vi "Create IO Channels Parallel.vi"(6 "AI Buffer Size (s)":i32=10, 8 "AI Block Size":i32=5000, 9 "Cluster":T1={"amplitude (V)"=[0.001, 2e-08, 0.001, 0.001, 0.001, 2e-08, 0.0, 0.0], "DC (V)"=[0.0, 0.0, 0.0, 0.0, 0.0, 0.0, 0.0, 0.0], "f (Hz)"=[13.0, 13.0, 13.0, 13.0, 13.0, 13.0, 13.0, 13.0], "phase (deg)"=[0.0, 0.0, 0.0, 0.0, 0.0, 0.0, 0.0, 0.0], "demod f (Hz)"=[13.0, 13.0, 13.0, 13.0, 13.0, 13.0, 13.0, 13.0], "function"=[enum."Sine Wave", enum."Sine Wave", enum."Sine Wave", enum."Sine Wave", enum."Sine Wave", enum."Sine Wave", enum."Sine Wave", enum."Sine Wave"]} {"DC (V)" format="%#_6p"; "amplitude (V)" format="%#_6p"}, 10 "AO Configuration":T2(array[cluster])=[{"Output physical channels"="PXI1Slot2/ao0", "AO. Max"=0.1, "AO.Min"=-0.1}, {"Output physical channels"="", "AO. Max"=0.1, "AO.Min"=-0.1}], 11 "AI Configuration":T3(array[cluster])=[{"AI.Coupling"=10050, "AI.Max"=10.0, "AI.Min"=-10.0, "Input physical channels"="PXI1Slot2/ai0:1"}, {"AI.Coupling"=10050, "AI.Max"=10.0, "AI.Min"=-10.0, "Input physical channels"="PXI1Slot3/ai0:3"}, {"AI.Coupling"=10050, "AI.Max"=10.0, "AI.Min"=-10.0, "Input physical channels"=""}] {"AI.Coupling" items=["AC"=10045, "DC"=10050, "GND"=10066]}) -> (0 "sampling info":cluster{"Fs":dbl, "#s":dbl}, 1 "AI Rate":dbl=10000.0 format="%.2f", 2 "AO Task":refnum<k21>[](array[refnum]), 3 "AI task":refnum<k21>[](array[refnum]), 4 "phase log":dbl[](array[numeric])=[0.99999999999938, 0.99999999999938], 5 "appended array":errorcluster[][](array[cluster]))   [LabVIEW 2013]
uses:
  <vilib>/DAQmx/write.llb/DAQmx Write (Analog 1D Wfm NChan NSamp).vi
  <vilib>/DAQmx/create/channels.llb/DAQmx Create Channel (AI-Voltage-Basic).vi
  <vilib>/DAQmx/create/channels.llb/DAQmx Create Channel (AO-Voltage-Basic).vi
  <vilib>/DAQmx/configure/timing.llb/DAQmx Timing (Sample Clock).vi
  <vilib>/DAQmx/configure/trigger.llb/DAQmx Start Trigger (Digital Edge).vi
  <vilib>/DAQmx/miscellaneous.llb/DAQmx Fill In Error Info.vi
  <resource>/objmgr/daqmx.rc
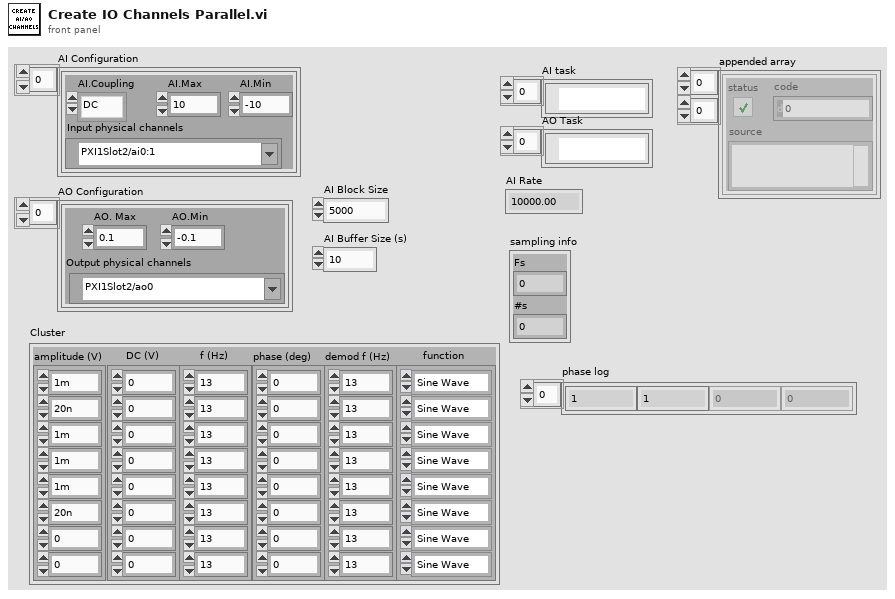
[diagram p1: front panel]
types:
  T1 = cluster{"amplitude (V)":dbl[], "DC (V)":dbl[], "f (Hz)":dbl[], "phase (deg)":dbl[], "demod f (Hz)":dbl[], "function":enum16{"Sine Wave", "Triangle Wave", "Square Wave", "Sawtooth Wave"}[]}
  T2 = cluster{"Output physical channels":tag, "AO. Max":dbl, "AO.Min":dbl}[]
  T3 = cluster{"AI.Coupling":i32, "AI.Max":dbl, "AI.Min":dbl, "Input physical channels":tag}[]
  T4 = cluster{"AI.Coupling":i32, "AI.Max":dbl, "AI.Min":dbl, "Input physical channels":tag}
  T5 = cluster{"Output physical channels":tag, "AO. Max":dbl, "AO.Min":dbl}
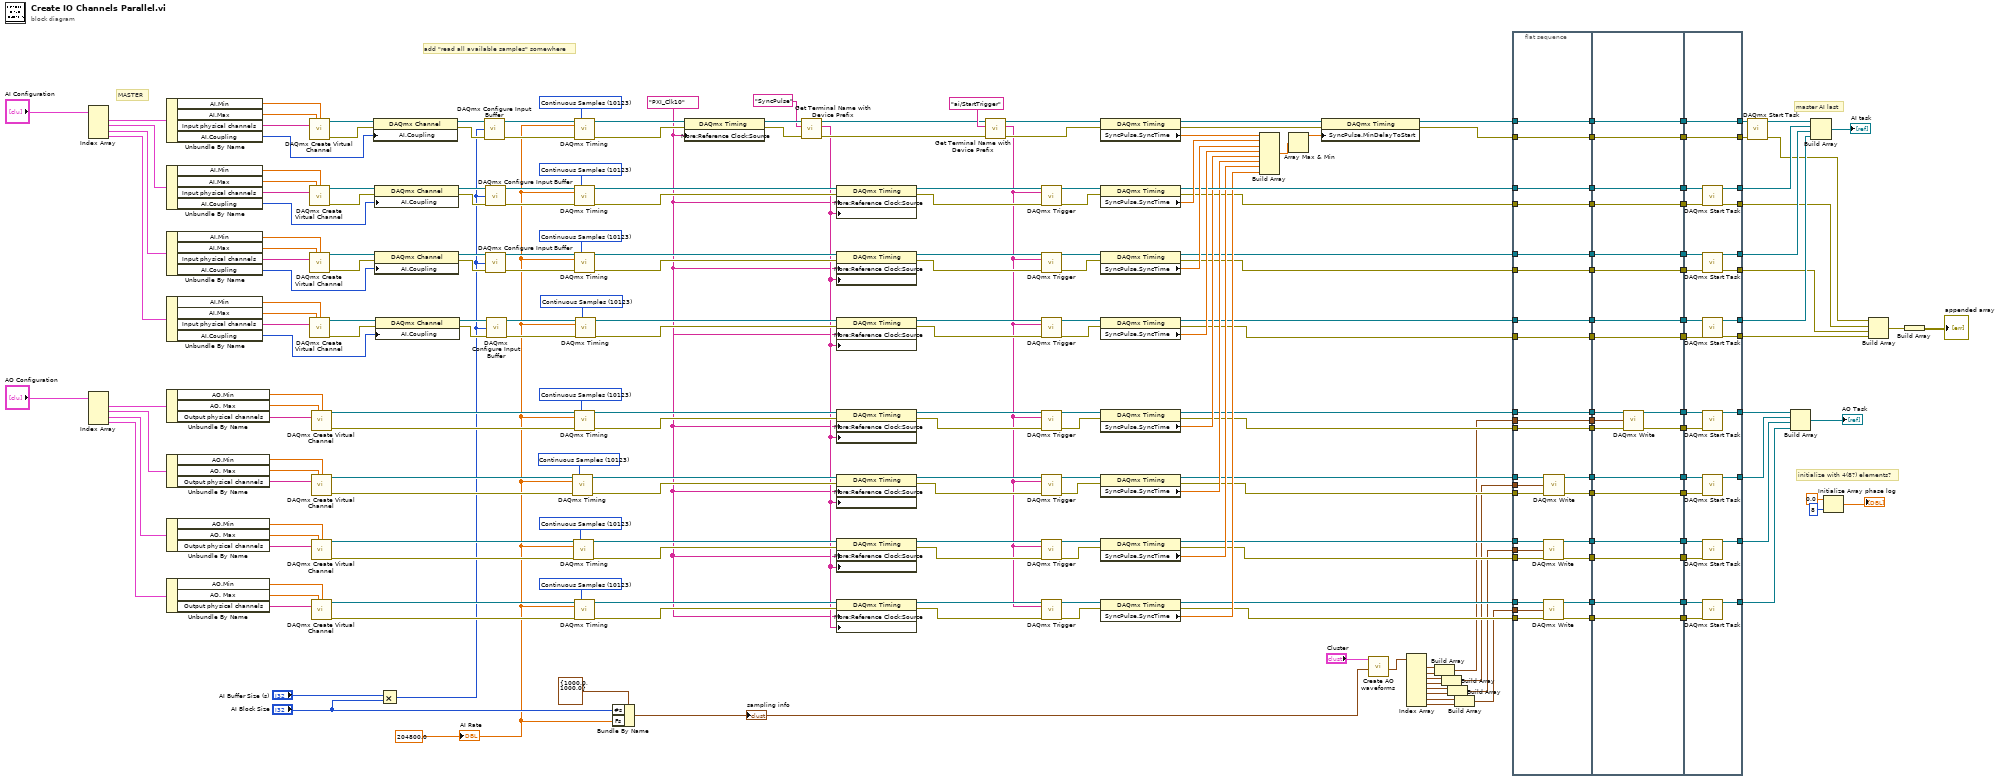
[diagram p0: block diagram]
diagram:
  w7 = 204800.0
  w23 = tag "PXI_Clk10" ("RefClk.Src")
  w96 = 10123 items=["Finite Samples"=10178, "Continuous Samples"=10123] ("sample mode")
  w111 = 10123 items=["Finite Samples"=10178, "Continuous Samples"=10123] ("sample mode")
  w120 = 10123 items=["Finite Samples"=10178, "Continuous Samples"=10123] ("sample mode")
  w134 = 10123 items=["Finite Samples"=10178, "Continuous Samples"=10123] ("sample mode")
  w161 = 10123 items=["Finite Samples"=10178, "Continuous Samples"=10123] ("sample mode")
  w177 = 10123 items=["Finite Samples"=10178, "Continuous Samples"=10123] ("sample mode")
  w190 = 10123 items=["Finite Samples"=10178, "Continuous Samples"=10123] ("sample mode")
  w230 = 10123 items=["Finite Samples"=10178, "Continuous Samples"=10123] ("sample mode")
  # "master AI last"
  # "initialize with 4(8?) elements?"
  # "add \"read all available samples\" somewhere"
  # "MASTER"
  n1 = Index Array(array="AI Configuration") -> (element #1=w231:T4, element #2=w191:T4, element #3=w154:T4, element #4=w153:T4)  [unwired: 4 in]
  n2 = Index Array(array="AO Configuration") -> (element #1=w138:T5, element #2=w89:T5, element #3=w90:T5, element #4=w91:T5)  [unwired: 4 in]
  n3 = Unbundle By Name(w231) -> ("AI.Min"=w202:dbl, "AI.Max"=w203:dbl, "Input physical channels"=w215:tag, "AI.Coupling"=w201:i32)
  n4 = Unbundle By Name(w191) -> ("AI.Min"=w198:dbl, "AI.Max"=w197:dbl, "Input physical channels"=w192:tag, "AI.Coupling"=w199:i32)
  n5 = Unbundle By Name(w154) -> ("AI.Min"=w170:dbl, "AI.Max"=w171:dbl, "Input physical channels"=w176:tag, "AI.Coupling"=w169:i32)
  n6 = Unbundle By Name(w153) -> ("AI.Min"=w167:dbl, "AI.Max"=w166:dbl, "Input physical channels"=w162:tag, "AI.Coupling"=w168:i32)
  n7 = Unbundle By Name(w138) -> ("AO.Min"=w135:dbl, "AO. Max"=w136:dbl, "Output physical channels"=w137:tag)
  n8 = Unbundle By Name(w89) -> ("AO.Min"=w118:dbl, "AO. Max"=w117:dbl, "Output physical channels"=w116:tag)
  n9 = Unbundle By Name(w90) -> ("AO.Min"=w113:dbl, "AO. Max"=w114:dbl, "Output physical channels"=w115:tag)
  n10 = Unbundle By Name(w91) -> ("AO.Min"=w94:dbl, "AO. Max"=w93:dbl, "Output physical channels"=w92:tag)
  n11 = call-poly <vilib>:"DAQmx Create Virtual Channel.vi"("maximum value"=w203, "minimum value"=w202, "physical channels"=w215) -> ("task out"=w214:refnum<k21>, "error out"=w213:errorcluster)  [unwired: 11 in]
  n12 = call-poly <vilib>:"DAQmx Create Virtual Channel.vi"("maximum value"=w197, "minimum value"=w198, "physical channels"=w192) -> ("task out"=w193:refnum<k21>, "error out"=w194:errorcluster)  [unwired: 11 in]
  n13 = call-poly <vilib>:"DAQmx Create Virtual Channel.vi"("maximum value"=w171, "minimum value"=w170, "physical channels"=w176) -> ("task out"=w175:refnum<k21>, "error out"=w174:errorcluster)  [unwired: 11 in]
  n14 = call-poly <vilib>:"DAQmx Create Virtual Channel.vi"("maximum value"=w166, "minimum value"=w167, "physical channels"=w162) -> ("task out"=w163:refnum<k21>, "error out"=w164:errorcluster)  [unwired: 11 in]
  n15 = call-poly <vilib>:"DAQmx Create Virtual Channel.vi"("maximum value"=w136, "minimum value"=w135, "physical channels"=w137) -> ("task out"=w21:refnum<k21>, "error out"=w20:errorcluster)  [unwired: 11 in]
  n16 = call-poly <vilib>:"DAQmx Create Virtual Channel.vi"("maximum value"=w117, "minimum value"=w118, "physical channels"=w116) -> ("task out"=w119:refnum<k21>, "error out"=w121:errorcluster)  [unwired: 11 in]
  n17 = call-poly <vilib>:"DAQmx Create Virtual Channel.vi"("maximum value"=w114, "minimum value"=w113, "physical channels"=w115) -> ("task out"=w112:refnum<k21>, "error out"=w110:errorcluster)  [unwired: 11 in]
  n18 = call-poly <vilib>:"DAQmx Create Virtual Channel.vi"("maximum value"=w93, "minimum value"=w94, "physical channels"=w92) -> ("task out"=w95:refnum<k21>, "error out"=w97:errorcluster)  [unwired: 11 in]
  n19 = property class="DAQmx Channel"(reference=w214, error in=w213, "AI.Coupling"=w201) -> (reference out=w212:refnum<k21>, error out=w211:errorcluster)
  n20 = property class="DAQmx Channel"(reference=w193, error in=w194, "AI.Coupling"=w199) -> (reference out=w195:refnum<k21>, error out=w196:errorcluster)
  n21 = property class="DAQmx Channel"(reference=w175, error in=w174, "AI.Coupling"=w169) -> (reference out=w173:refnum<k21>, error out=w172:errorcluster)
  n22 = property class="DAQmx Channel"(reference=w163, error in=w164, "AI.Coupling"=w168) -> (reference out=w165:refnum<k21>, error out=w28:errorcluster)
  n23 = Multiply(x="AI Buffer Size (s)", y="AI Block Size") -> (x*y=w4:i32)
  n24 = call <vilib>:"DAQmx Configure Input Buffer.vi"("task/channels in"=w212, "buffer size (in samples per channel)"=w4, "error in"=w211) -> ("task out"=w210:refnum<k21>, "error out"=w209:errorcluster)  [unwired: 11 in]
  n25 = call <vilib>:"DAQmx Configure Input Buffer.vi"("task/channels in"=w195, "buffer size (in samples per channel)"=w4, "error in"=w196) -> ("task out"=w189:refnum<k21>, "error out"=w188:errorcluster)  [unwired: 11 in]
  n26 = call <vilib>:"DAQmx Configure Input Buffer.vi"("task/channels in"=w173, "buffer size (in samples per channel)"=w4, "error in"=w172) -> ("task out"=w178:refnum<k21>, "error out"=w179:errorcluster)  [unwired: 11 in]
  n27 = call <vilib>:"DAQmx Configure Input Buffer.vi"("task/channels in"=w165, "buffer size (in samples per channel)"=w4, "error in"=w28) -> ("task out"=w160:refnum<k21>, "error out"=w159:errorcluster)  [unwired: 11 in]
  n28 = call-poly <vilib>:"DAQmx Timing.vi"("task/channels in"=w119, "sample mode"=w120, "rate"=w7, "error in"=w121) -> ("task out"=w123:refnum<k21>, "error out"=w124:errorcluster)  [unwired: 10 in]
  n29 = call-poly <vilib>:"DAQmx Timing.vi"("task/channels in"=w112, "sample mode"=w111, "rate"=w7, "error in"=w110) -> ("task out"=w108:refnum<k21>, "error out"=w107:errorcluster)  [unwired: 10 in]
  n30 = call-poly <vilib>:"DAQmx Timing.vi"("task/channels in"=w210, "sample mode"=w230, "rate"=w7, "error in"=w209) -> ("task out"=w229:refnum<k21>, "error out"=w200:errorcluster)  [unwired: 10 in]
  n31 = call-poly <vilib>:"DAQmx Timing.vi"("task/channels in"=w189, "sample mode"=w190, "rate"=w7, "error in"=w188) -> ("task out"=w187:refnum<k21>, "error out"=w186:errorcluster)  [unwired: 10 in]
  n32 = call-poly <vilib>:"DAQmx Timing.vi"("task/channels in"=w178, "sample mode"=w177, "rate"=w7, "error in"=w179) -> ("task out"=w180:refnum<k21>, "error out"=w181:errorcluster)  [unwired: 10 in]
  n33 = call-poly <vilib>:"DAQmx Timing.vi"("task/channels in"=w21, "sample mode"=w134, "rate"=w7, "error in"=w20) -> ("task out"=w132:refnum<k21>, "error out"=w131:errorcluster)  [unwired: 10 in]
  n34 = call-poly <vilib>:"DAQmx Timing.vi"("task/channels in"=w95, "sample mode"=w96, "rate"=w7, "error in"=w97) -> ("task out"=w99:refnum<k21>, "error out"=w100:errorcluster)  [unwired: 10 in]
  n35 = call-poly <vilib>:"DAQmx Timing.vi"("task/channels in"=w160, "sample mode"=w161, "rate"=w7, "error in"=w159) -> ("task out"=w158:refnum<k21>, "error out"=w157:errorcluster)  [unwired: 10 in]
  n36 = Bundle By Name(cluster=cluster{"Fs":dbl, "#s":dbl} {"Fs"=1000.0, "#s"=1000.0} ("sampling info"), "#s"="AI Block Size", "Fs"=w7) -> (w6:cluster{"Fs":dbl, "#s":dbl})
  "sampling info" <- w6
  n37 = property class="DAQmx Timing"(reference=w229, error in=w200, "More:Reference Clock:Source"=w23) -> (reference out=w27:refnum<k21>, error out=w26:errorcluster)
  n38 = call "Get Terminal Name with Device Prefix.vi"("error in (no error)"=w26, "Local Terminal Name"="SyncPulse", "task/channels in"=w27) -> ("error out"=w224:errorcluster, "Terminal Name with Device Prefix"=w24:tag, "task out"=w225:refnum<k21>)  [unwired: 6 in]
  n39 = property class="DAQmx Timing"(reference=w187, error in=w186, "More:Reference Clock:Source"=w23, "More:Synchronization Pulse:Source"=w24) -> (reference out=w185:refnum<k21>, error out=w184:errorcluster)
  n40 = property class="DAQmx Timing"(reference=w180, error in=w181, "More:Reference Clock:Source"=w23, "More:Synchronization Pulse:Source"=w24) -> (reference out=w182:refnum<k21>, error out=w183:errorcluster)
  n41 = property class="DAQmx Timing"(reference=w158, error in=w157, "More:Reference Clock:Source"=w23, "More:Synchronization Pulse:Source"=w24) -> (reference out=w156:refnum<k21>, error out=w155:errorcluster)
  n42 = property class="DAQmx Timing"(reference=w132, error in=w131, "More:Reference Clock:Source"=w23, "More:Synchronization Pulse:Source"=w24) -> (reference out=w133:refnum<k21>, error out=w130:errorcluster)
  n43 = property class="DAQmx Timing"(reference=w123, error in=w124, "More:Reference Clock:Source"=w23, "More:Synchronization Pulse:Source"=w24) -> (reference out=w122:refnum<k21>, error out=w125:errorcluster)
  n44 = property class="DAQmx Timing"(reference=w108, error in=w107, "More:Reference Clock:Source"=w23, "More:Synchronization Pulse:Source"=w24) -> (reference out=w109:refnum<k21>, error out=w106:errorcluster)
  n45 = property class="DAQmx Timing"(reference=w99, error in=w100, "More:Reference Clock:Source"=w23, "More:Synchronization Pulse:Source"=w24) -> (reference out=w98:refnum<k21>, error out=w101:errorcluster)
  n46 = call "Get Terminal Name with Device Prefix.vi"("error in (no error)"=w224, "Local Terminal Name"="ai/StartTrigger", "task/channels in"=w225) -> ("error out"=w222:errorcluster, "Terminal Name with Device Prefix"=w84:tag, "task out"=w223:refnum<k21>)  [unwired: 6 in]
  n47 = call-poly <vilib>:"DAQmx Trigger.vi"("task/channels in"=w185, "source"=w84, "error in"=w184) -> ("task out"=w150:refnum<k21>, "error out"=w149:errorcluster)  [unwired: 11 in]
  n48 = call-poly <vilib>:"DAQmx Trigger.vi"("task/channels in"=w182, "source"=w84, "error in"=w183) -> ("task out"=w151:refnum<k21>, "error out"=w148:errorcluster)  [unwired: 11 in]
  n49 = call-poly <vilib>:"DAQmx Trigger.vi"("task/channels in"=w156, "source"=w84, "error in"=w155) -> ("task out"=w152:refnum<k21>, "error out"=w147:errorcluster)  [unwired: 11 in]
  n50 = call-poly <vilib>:"DAQmx Trigger.vi"("task/channels in"=w133, "source"=w84, "error in"=w130) -> ("task out"=w129:refnum<k21>, "error out"=w128:errorcluster)  [unwired: 11 in]
  n51 = call-poly <vilib>:"DAQmx Trigger.vi"("task/channels in"=w122, "source"=w84, "error in"=w125) -> ("task out"=w126:refnum<k21>, "error out"=w127:errorcluster)  [unwired: 11 in]
  n52 = call-poly <vilib>:"DAQmx Trigger.vi"("task/channels in"=w109, "source"=w84, "error in"=w106) -> ("task out"=w105:refnum<k21>, "error out"=w104:errorcluster)  [unwired: 11 in]
  n53 = call-poly <vilib>:"DAQmx Trigger.vi"("task/channels in"=w98, "source"=w84, "error in"=w101) -> ("task out"=w102:refnum<k21>, "error out"=w103:errorcluster)  [unwired: 11 in]
  n54 = property class="DAQmx Timing"(reference=w223, error in=w222) -> (reference out=w219:refnum<k21>, error out=w220:errorcluster, "SyncPulse.SyncTime"=w221:dbl)
  n55 = property class="DAQmx Timing"(reference=w150, error in=w149) -> (reference out=w140:refnum<k21>, error out=w75:errorcluster, "SyncPulse.SyncTime"=w145:dbl)
  n56 = property class="DAQmx Timing"(reference=w151, error in=w148) -> (reference out=w81:refnum<k21>, error out=w72:errorcluster, "SyncPulse.SyncTime"=w144:dbl)
  n57 = property class="DAQmx Timing"(reference=w152, error in=w147) -> (reference out=w78:refnum<k21>, error out=w69:errorcluster, "SyncPulse.SyncTime"=w143:dbl)
  n58 = property class="DAQmx Timing"(reference=w129, error in=w128) -> (reference out=w66:refnum<k21>, error out=w57:errorcluster, "SyncPulse.SyncTime"=w88:dbl)
  n59 = property class="DAQmx Timing"(reference=w126, error in=w127) -> (reference out=w63:refnum<k21>, error out=w55:errorcluster, "SyncPulse.SyncTime"=w87:dbl)
  n60 = property class="DAQmx Timing"(reference=w105, error in=w104) -> (reference out=w60:refnum<k21>, error out=w52:errorcluster, "SyncPulse.SyncTime"=w86:dbl)
  n61 = property class="DAQmx Timing"(reference=w102, error in=w103) -> (reference out=w49:refnum<k21>, error out=w46:errorcluster, "SyncPulse.SyncTime"=w85:dbl)
  n62 = Build Array(w221, w145, w144, w143, w88, w87, w86, w85) -> (w218:dbl[])
  n63 = Array Max & Min(array=w218) -> (max value=w146:dbl)  [unwired: 3 out]
  n64 = property class="DAQmx Timing"(reference=w219, error in=w220, "SyncPulse.MinDelayToStart"=w146) -> (reference out=w216:refnum<k21>, error out=w217:errorcluster)
  n65 = call "Create AO waveforms.vi"("sampling info"=w6, "Cluster"="Cluster") -> ("AO Array"=w1:waveform(dbl)[])  [unwired: 8 in, 1 out]
  n66 = Index Array(array=w1) -> (element #1=w8:waveform(dbl), element #2=w19:waveform(dbl), element #3=w18:waveform(dbl), element #4=w17:waveform(dbl), element #5=w16:waveform(dbl), element #6=w15:waveform(dbl), element #7=w14:waveform(dbl), element #8=w13:waveform(dbl))  [unwired: 8 in]
  n67 = Build Array(w8, w19) -> (w12:waveform(dbl)[])
  n68 = Build Array(w18, w17) -> (w11:waveform(dbl)[])
  n69 = Build Array(w16, w15) -> (w10:waveform(dbl)[])
  n70 = Build Array(w14, w13) -> (w9:waveform(dbl)[])
  n71 = flat-sequence {
    tunnel: w217 -> [w260]
    tunnel: w216 -> [w261]
    tunnel: [w261] -> w235
    tunnel: [w260] -> w234
    tunnel: [w259] -> w141
    tunnel: w140 -> [w259]
    tunnel: [w258] -> w82
    tunnel: w81 -> [w258]
    tunnel: [w257] -> w79
    tunnel: w78 -> [w257]
    tunnel: [w256] -> w76
    tunnel: w75 -> [w256]
    tunnel: [w255] -> w73
    tunnel: w72 -> [w255]
    tunnel: [w254] -> w70
    tunnel: w69 -> [w254]
    tunnel: [w253] -> w67
    tunnel: w66 -> [w253]
    tunnel: [w241] -> w64
    tunnel: w63 -> [w242]
    tunnel: [w245] -> w61
    tunnel: w60 -> [w244]
    tunnel: [w252] -> w58
    tunnel: w57 -> [w252]
    tunnel: w55 -> [w243]
    tunnel: [w246] -> w53
    tunnel: w52 -> [w247]
    tunnel: [w248] -> w50
    tunnel: w49 -> [w251]
    tunnel: [w249] -> w47
    tunnel: w46 -> [w250]
    tunnel: [w240] -> w45
    tunnel: [w239] -> w36
    tunnel: w12 -> [w239]
    tunnel: w11 -> [w238]
    tunnel: w10 -> [w237]
    tunnel: w9 -> [w236]
    tunnel: [w280] -> w233
    tunnel: [w279] -> w232
    tunnel: w235 -> [w280]
    tunnel: w234 -> [w279]
    tunnel: [w278] -> w142
    tunnel: w141 -> [w278]
    tunnel: [w277] -> w83
    tunnel: w82 -> [w277]
    tunnel: [w276] -> w80
    tunnel: w79 -> [w276]
    tunnel: [w275] -> w77
    tunnel: w76 -> [w275]
    tunnel: [w274] -> w74
    tunnel: w73 -> [w274]
    tunnel: [w273] -> w71
    tunnel: w70 -> [w273]
    tunnel: [w265] -> w68
    tunnel: w67 -> [w266]
    tunnel: [w272] -> w65
    tunnel: w64 -> [w272]
    tunnel: [w271] -> w62
    tunnel: w61 -> [w271]
    tunnel: [w264] -> w59
    tunnel: w58 -> [w263]
    tunnel: [w270] -> w56
    tunnel: [w269] -> w54
    tunnel: w53 -> [w269]
    tunnel: [w268] -> w51
    tunnel: w50 -> [w268]
    tunnel: [w267] -> w48
    tunnel: w47 -> [w267]
    tunnel: w45 -> [w270]
    tunnel: w36 -> [w262]
    tunnel: [w306] -> w228
    tunnel: [w305] -> w227
    tunnel: w233 -> [w306]
    tunnel: w232 -> [w305]
    tunnel: w142 -> [w304]
    tunnel: w83 -> [w303]
    tunnel: w80 -> [w302]
    tunnel: w77 -> [w301]
    tunnel: w74 -> [w300]
    tunnel: w71 -> [w299]
    tunnel: w68 -> [w298]
    tunnel: w65 -> [w297]
    tunnel: w62 -> [w296]
    tunnel: w59 -> [w295]
    tunnel: w56 -> [w294]
    tunnel: w54 -> [w293]
    tunnel: w51 -> [w292]
    tunnel: w48 -> [w291]
    tunnel: [w290] -> w44
    tunnel: [w289] -> w43
    tunnel: [w288] -> w42
    tunnel: [w287] -> w41
    tunnel: [w286] -> w40
    tunnel: [w285] -> w39
    tunnel: [w284] -> w38
    tunnel: [w283] -> w35
    tunnel: [w282] -> w32
    tunnel: [w281] -> w34
    frame #0 {
      n72 = call-poly <vilib>:"DAQmx Write.vi"("task/channels in"=w244, "data"=w237, "error in"=w247) -> ("task out"=w245:refnum<k21>, "error out"=w246:errorcluster)  [unwired: 10 in, 1 out]
      n73 = call-poly <vilib>:"DAQmx Write.vi"("task/channels in"=w251, "data"=w236, "error in"=w250) -> ("task out"=w248:refnum<k21>, "error out"=w249:errorcluster)  [unwired: 10 in, 1 out]
      n74 = call-poly <vilib>:"DAQmx Write.vi"("task/channels in"=w242, "data"=w238, "error in"=w243) -> ("task out"=w241:refnum<k21>, "error out"=w240:errorcluster)  [unwired: 10 in, 1 out]
    }
    frame #1 {
      n75 = call-poly <vilib>:"DAQmx Write.vi"("task/channels in"=w266, "data"=w262, "error in"=w263) -> ("task out"=w265:refnum<k21>, "error out"=w264:errorcluster)  [unwired: 10 in, 1 out]
    }
    frame #2 {
      n76 = call <vilib>:"DAQmx Start Task.vi"("task/channels in"=w304, "error in"=w301) -> ("task out"=w290:refnum<k21>, "error out"=w283:errorcluster)  [unwired: 12 in]
      n77 = call <vilib>:"DAQmx Start Task.vi"("task/channels in"=w303, "error in"=w300) -> ("task out"=w289:refnum<k21>, "error out"=w282:errorcluster)  [unwired: 12 in]
      n78 = call <vilib>:"DAQmx Start Task.vi"("task/channels in"=w302, "error in"=w299) -> ("task out"=w288:refnum<k21>, "error out"=w281:errorcluster)  [unwired: 12 in]
      n79 = call <vilib>:"DAQmx Start Task.vi"("task/channels in"=w298, "error in"=w295) -> ("task out"=w287:refnum<k21>)  [unwired: 12 in, 1 out]
      n80 = call <vilib>:"DAQmx Start Task.vi"("task/channels in"=w297, "error in"=w294) -> ("task out"=w286:refnum<k21>)  [unwired: 12 in, 1 out]
      n81 = call <vilib>:"DAQmx Start Task.vi"("task/channels in"=w296, "error in"=w293) -> ("task out"=w285:refnum<k21>)  [unwired: 12 in, 1 out]
      n82 = call <vilib>:"DAQmx Start Task.vi"("task/channels in"=w292, "error in"=w291) -> ("task out"=w284:refnum<k21>)  [unwired: 12 in, 1 out]
    }
  }
  n83 = call <vilib>:"DAQmx Start Task.vi"("task/channels in"=w228, "error in"=w227) -> ("task out"=w207:refnum<k21>, "error out"=w22:errorcluster)  [unwired: 12 in]
  n84 = Build Array(w41, w40, w39, w38) -> (→"AO Task":refnum<k21>[])
  n85 = Build Array(w207, w44, w43, w42) -> (→"AI task":refnum<k21>[])
  n86 = Initialize Array(0.0 ("element"), 8 ("dimension size")) -> (→"phase log":dbl[])
  n87 = Build Array(w22, w35, w32, w34) -> (w33:errorcluster[])
  n88 = Build Array(w33) -> (→"appended array":errorcluster[][])
  "AI Rate" <- w7
